vi "Display Prop 3.vi"(11 "GIC Input":T1={"     Use ?\nOff       On"=[FALSE, TRUE, FALSE, TRUE], "Mode:"=FALSE, "Rx Prop Port"="", "Hokuyo Port"="COM7", "Tx Prop  Port"="COM6", "Compass Port"="", "GPS Port"="", "Num of WPs"=0, "WP Lats and Longs"={"WP Lats"=[], "WP Longs"=[]}, "Obst Lats and Longs"={"Obst Lats"=[], "Obst Longs"=[]}, "Parameters"=[], "GPS Data"=[], "Compass"=0.0, "LMS Vector"=[], "Vision Vector"=[], "Direction Cmd"=0.0, "Speed Cmd"=0.0, "WP Vector"=[], "WP Number"=0, "Extra"=0, "SW Map"=[], "Path Cluster"={"Path x node"=[], "Path y node"=[]}} {"Obst Lats and Longs"."Obst Longs" format="%#_8g"; "Obst Lats and Longs"."Obst Lats" format="%#_8g"}) -> (1 "?":string, 2 "Right/Left":dbl, 3 "Forward/Reverse":dbl)   [LabVIEW 2014]
uses:
  <vilib>/Instr/_visa.llb/VISA Configure Serial Port (Instr).vi
panel:
  # "Display Prop 3"
  # "Input:"
  # "Output:"
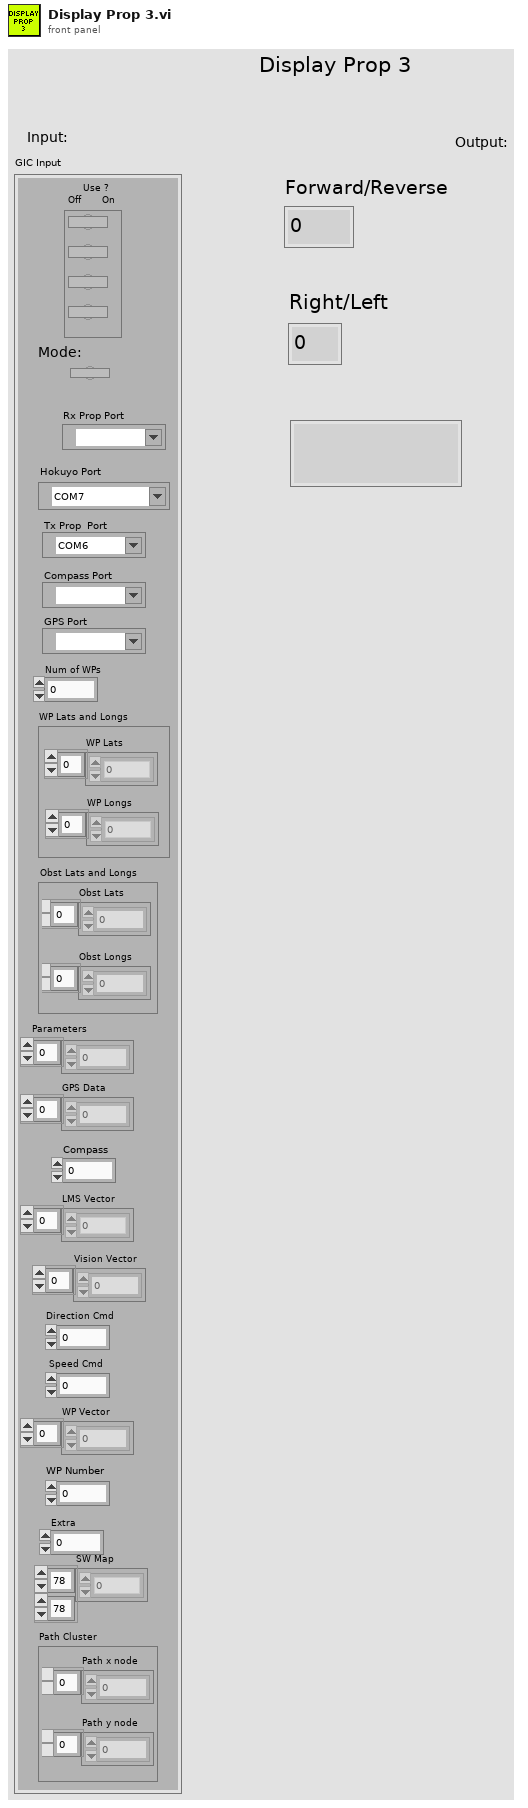
[diagram p1: front panel]
types:
  T1 = cluster{"     Use ?\nOff       On":bool[], "Mode:":bool, "Rx Prop Port":refnum<visa-resource-name>, "Hokuyo Port":refnum<visa-resource-name>, "Tx Prop  Port":refnum<visa-resource-name>, "Compass Port":refnum<visa-resource-name>, "GPS Port":refnum<visa-resource-name>, "Num of WPs":i16, "WP Lats and Longs":cluster{"WP Lats":dbl[], "WP Longs":dbl[]}, "Obst Lats and Longs":cluster{"Obst Lats":dbl[], "Obst Longs":dbl[]}, "Parameters":dbl[], "GPS Data":dbl[], "Compass":dbl, "LMS Vector":dbl[], "Vision Vector":dbl[], "Direction Cmd":dbl, "Speed Cmd":dbl, "WP Vector":dbl[], "WP Number":i32, "Extra":i16, "SW Map":i32[][], "Path Cluster":cluster{"Path x node":dbl[], "Path y node":dbl[]}}
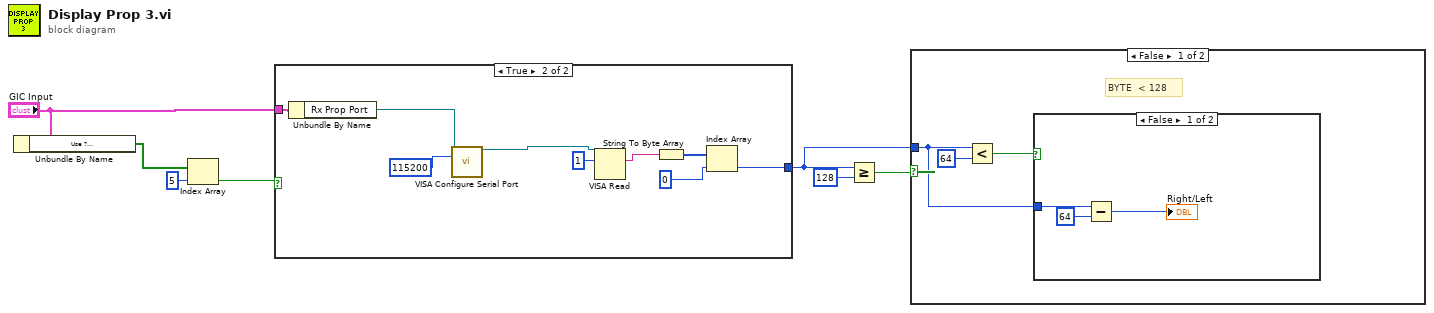
[diagram p0: block diagram]
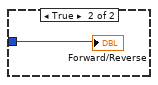
[diagram p2: hidden frame]
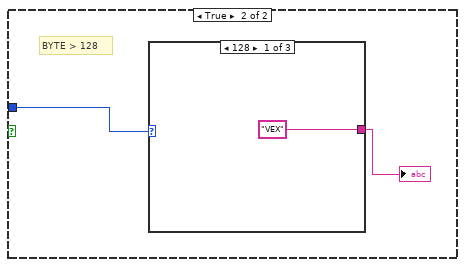
[diagram p3: hidden frame]
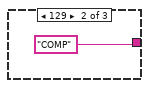
[diagram p4: hidden frame]
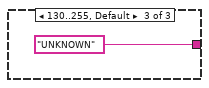
[diagram p5: hidden frame]
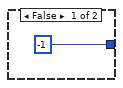
[diagram p6: hidden frame]
diagram:
  n1 = Unbundle By Name("GIC Input") -> ("Use ?\nOff       On"=w6:bool[])
  n2 = Index Array(array=w6, index=5) -> (element=w4:bool)
  n3 = case shown="True" w4 {
    tunnel: "GIC Input" -> [_ w17]
    tunnel: [-1 w10] -> w1
    frame False {
    }
    frame True {
      n4 = Unbundle By Name(w17) -> ("Rx Prop Port"=w16:refnum<visa-resource-name>)
      n5 = call-poly "VISA Configure Serial Port"("VISA resource name"=w16, "baud rate (9600)"=u32 115200) -> ("VISA resource name out"=w9:refnum<visa-resource-name>)  [unwired: 12 in, 1 out]
      n6 = VISA Read(VISA resource name=w9, byte count=u32 1) -> (read buffer=w11:string)  [unwired: 1 in, 3 out]
      n7 = String To Byte Array(string=w11) -> (unsigned byte array=w12:u8[])
      n8 = Index Array(array=w12, index=0) -> (element=w10:u8)
    }
  }
  n9 = Greater Or Equal?(x=w1, y=128) -> (x >= y?=w2:bool)
  n10 = case shown="False" w2 {
    tunnel: w1 -> [w18 w26]
    frame False {
      # "BYTE  < 128"
      n11 = Less?(x=w18, y=64) -> (x < y?=w19:bool)
      n12 = case shown="False" w19 {
        tunnel: w18 -> [w23 w24]
        frame False {
          n13 = Subtract(x=w23, y=64) -> (x-y=→"Right/Left":i32)
        }
        frame True {
          "Forward/Reverse" <- w24
        }
      }
    }
    frame True {
      # "BYTE > 128"
      n14 = case shown="128" w26 {
        tunnel: ["VEX" "COMP" "UNKNOWN"] -> w25
        frame 128 {
        }
        frame 129 {
        }
        frame 130..255, Default {
        }
      }
      "?" <- w25
    }
  }
